vi "CheckHandle.vi"(8 "error in (no error)":errorcluster, 10 "Connection Array":T1, 11 "Handle":string) -> (0 "error out":errorcluster, 2 "Instrument handle":refnum<k15>, 3 "Open Connection (F=Open)":bool)   [LabVIEW 2018, in "ScopePlugins.lvlib" / "NIScope.lvclass"]
doc: "Checks the name used to connect the instrument and reduces repeated connections."
uses:
  NIScope.lvclass
  ConnectionArray.ctl
  ScopePlugins.lvlib
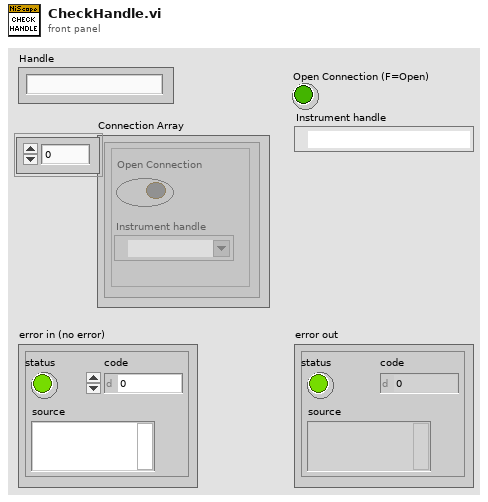
[diagram p1: front panel]
types:
  T1 = typedef "ScopePlugins.lvlib/ConnectionArray.ctl" = cluster{"Open Connection":bool, "Instrument handle":refnum<k15>}[]
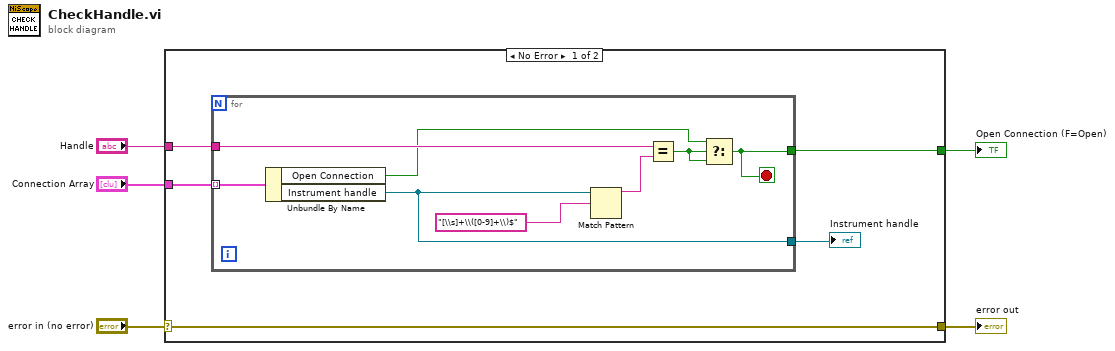
[diagram p0: block diagram]
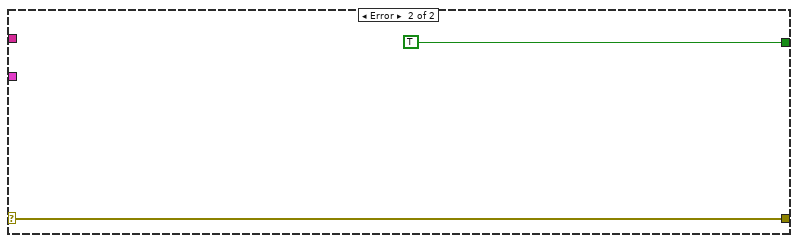
[diagram p2: hidden frame]
diagram:
  n1 = case shown="No Error" "error in (no error)" {
    selector: "error in (no error)" -> [w10 w20]
    tunnel: [w10 w20] -> w4
    tunnel: "Connection Array" -> [w6 _]
    tunnel: "Handle" -> [w9 _]
    tunnel: [w8 TRUE] -> w2
    frame No Error {
      n2 = for {
        tunnel: w9 -> [w16]
        tunnel: [w15] -> w8
        tunnel: w6 -> [w14] mode=indexing
        tunnel: [w12] -> w7
        stop <- w15 stop-if-true
        n3 = Unbundle By Name(w14) -> ("Open Connection"=w13:bool, "Instrument handle"=w12:refnum<k15>)
        n4 = Match Pattern(string=w12, regular expression="[\\s]+\\([0-9]+\\)$") -> (before substring=w17:string)  [unwired: 1 in, 3 out]
        n5 = Equal?(x=w16, y=w17) -> (x = y?=w11:bool)
        n6 = Select(t=w13, s=w11, f=w11) -> (s? t:f=w15:bool)
      }
      "Instrument handle" <- w7
    }
    frame Error {
    }
  }
  "error out" <- w4
  "Open Connection (F=Open)" <- w2
